vi "Autonomous Global.vi"() -> ()   [LabVIEW 2015]
uses:
  Play Info.ctl
panel:
  in  "Turn Error":dbl
  out "Autonomous Plays":T1[](array[typedef])
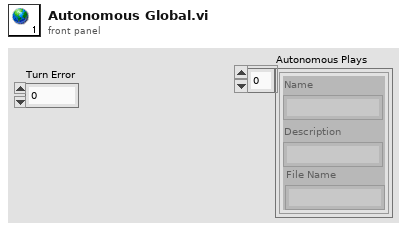
[diagram p1: front panel]
types:
  T1 = typedef "Play Info.ctl" = cluster{"Name":string, "Description":string, "File Name":string}
diagram:
